vi "measurement_loop_template.vi"(8 "error in (no error)":errorcluster, 9 "Hardware.lvclass":refnum<class "Hardware.lvclass">, 10 "Notifiers":T2, 11 "Message Queues":T1) -> (0 "error out":errorcluster)   [LabVIEW 2017]
uses:
  Notifiers/Notifiers.ctl
  Message Queue/All Message Queues.ctl
  Message Queue/Message Cluster.ctl
  hardware/Hardware.lvclass
  measurement_state.ctl
  Message Queue/Enqueue Message (Single).vi
  <vilib>/Utility/error.llb/Error Cluster From Error Code.vi
  <vilib>/ErrorRing/Error Ring.xnode
  Message Queue/Message Queue.lvlib
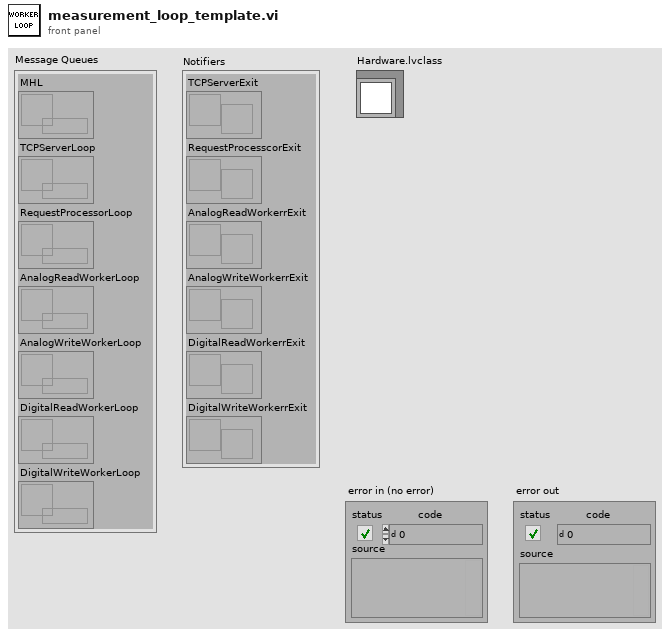
[diagram p1: front panel]
types:
  T1 = typedef "Message Queue.lvlib/All Message Queues.ctl" = cluster{"MHL":refnum<queue>, "TCPServerLoop":refnum<queue>, "RequestProcessorLoop":refnum<queue>, "AnalogReadWorkerLoop":refnum<queue>, "AnalogWriteWorkerLoop":refnum<queue>, "DigitalReadWorkerLoop":refnum<queue>, "DigitalWriteWorkerLoop":refnum<queue>}
  T2 = typedef "Notifiers.ctl" = cluster{"TCPServerExit":refnum<notifier>, "RequestProcesscorExit":refnum<notifier>, "AnalogReadWorkerrExit":refnum<notifier>, "AnalogWriteWorkerrExit":refnum<notifier>, "DigitalReadWorkerrExit":refnum<notifier>, "DigitalWriteWorkerrExit":refnum<notifier>}
  T3 = typedef "measurement_state.ctl" = enum16{"idle", "running"}
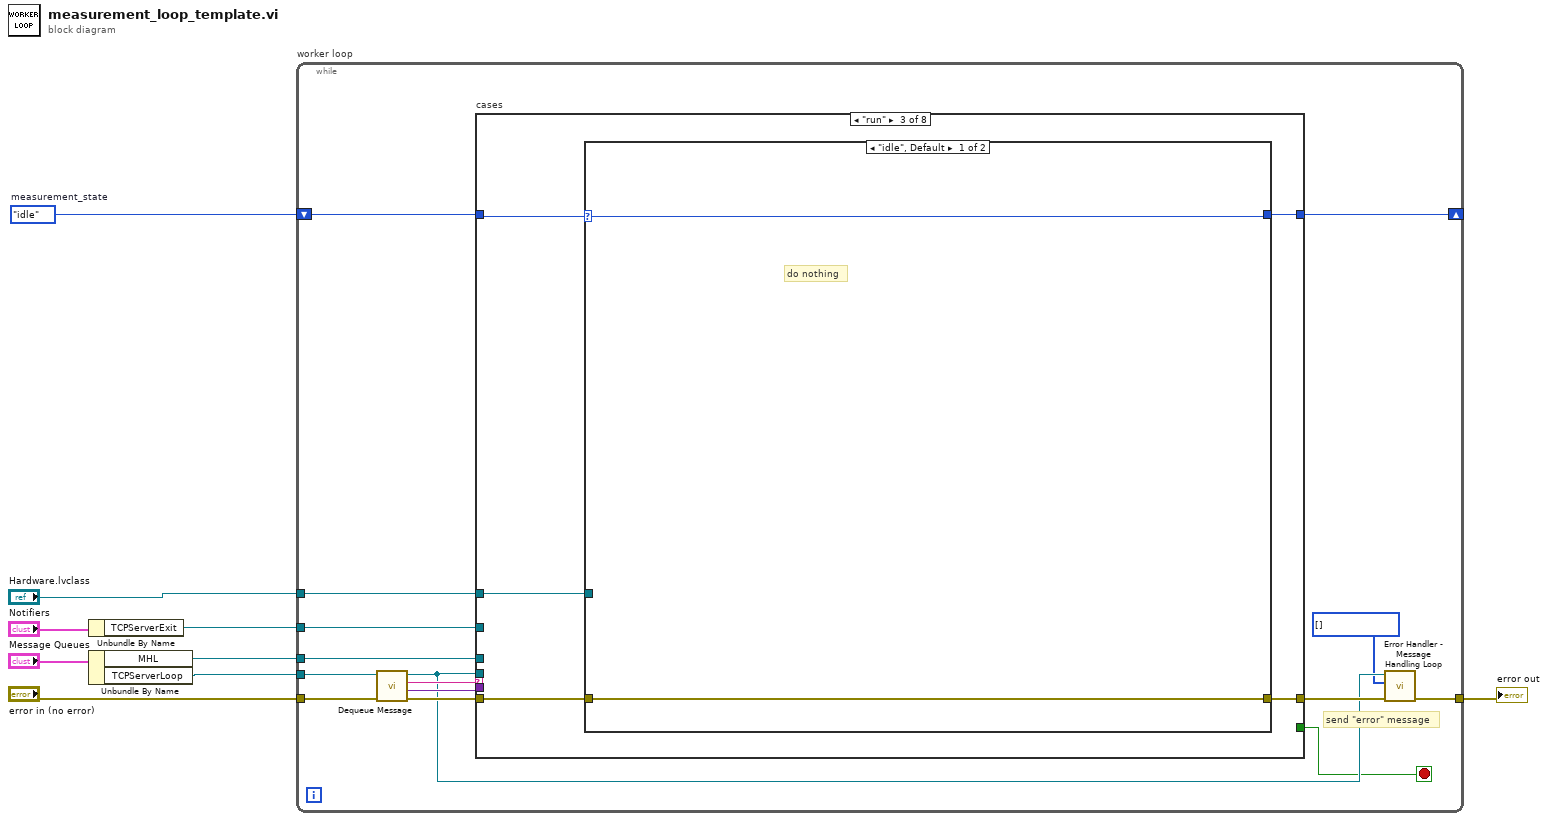
[diagram p0: block diagram]
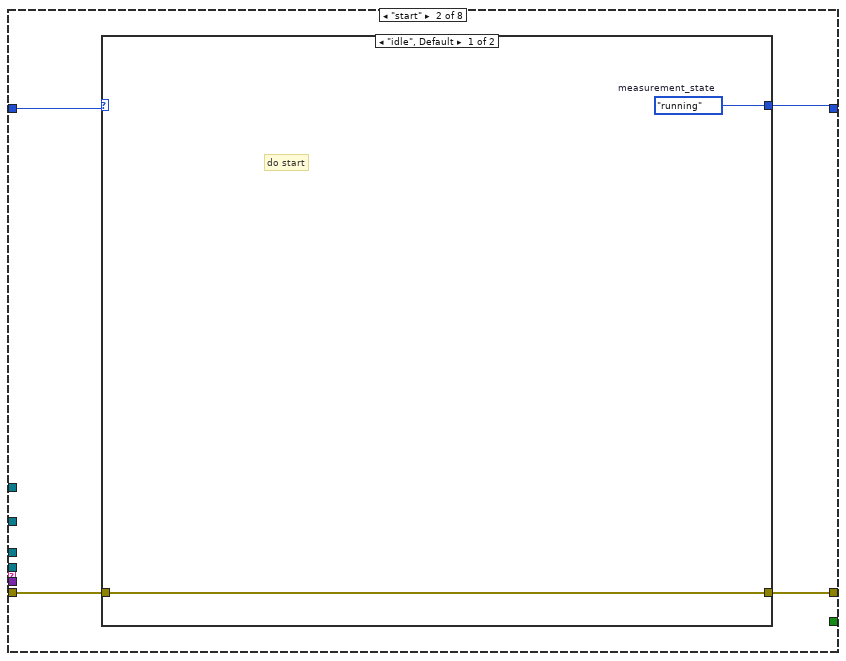
[diagram p3: hidden frame]
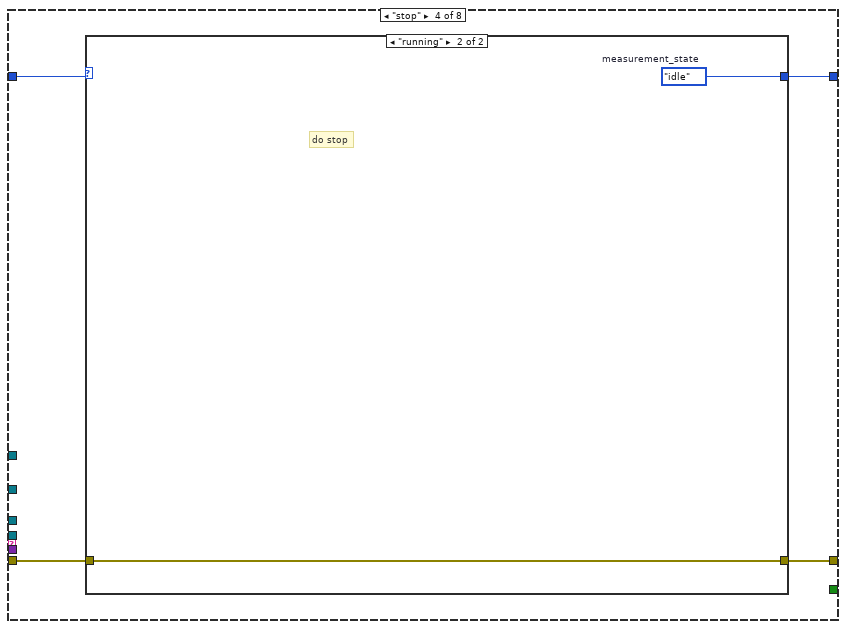
[diagram p6: hidden frame]
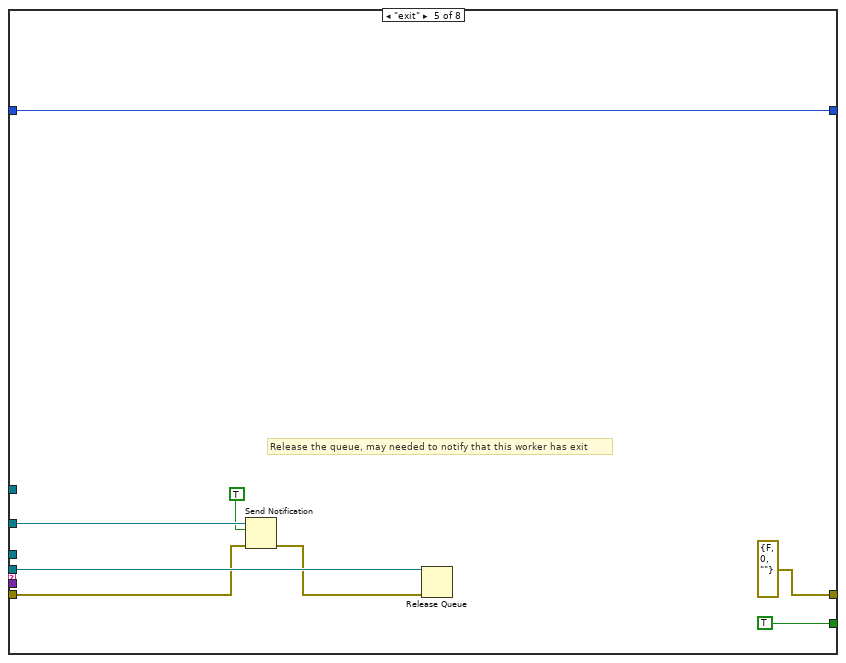
[diagram p8: hidden frame]
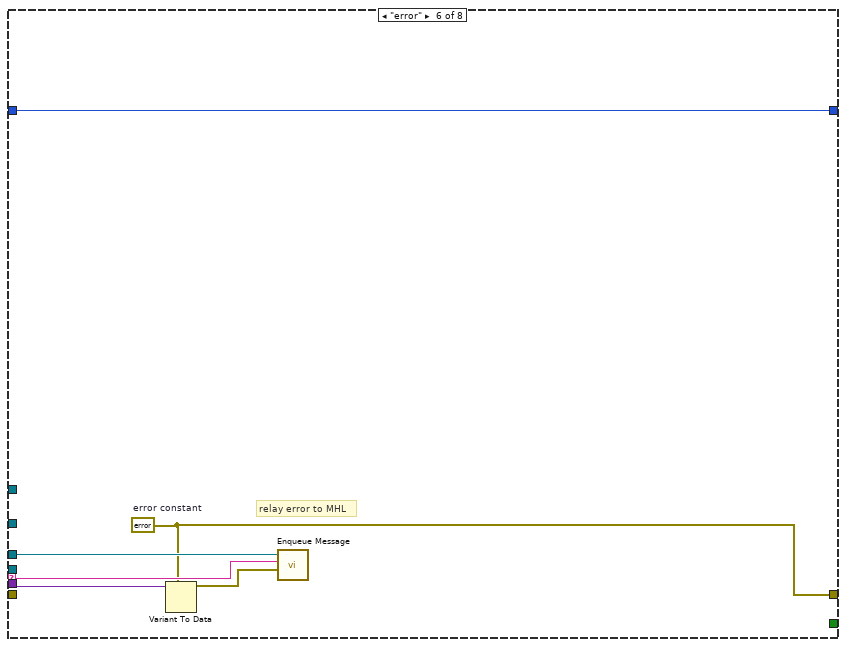
[diagram p9: hidden frame]
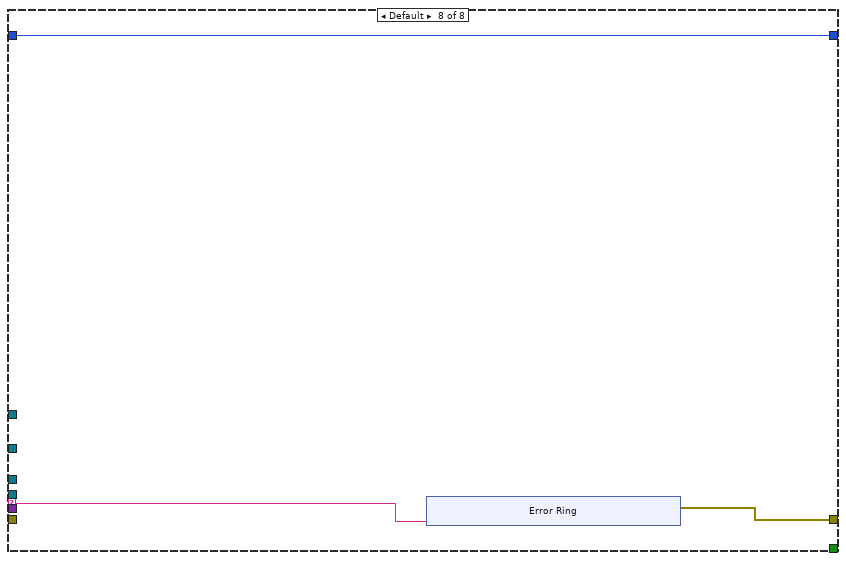
[diagram p11: hidden frame]
diagram:
  w1 = measurement_state."idle"  # measurement_state
  n1 = Unbundle By Name("Notifiers") -> ("TCPServerExit"=w3:refnum<notifier>)
  n2 = Unbundle By Name("Message Queues") -> ("MHL"=w5:refnum<queue>, "TCPServerLoop"=w6:refnum<queue>)
  n3 = while "worker loop" {
    tunnel: "error in (no error)" -> [w24]
    tunnel: [w19] -> w8
    tunnel: w6 -> [w15]
    tunnel: w5 -> [w14]
    tunnel: w3 -> [w13]
    tunnel: "Hardware.lvclass" -> [w12]
    shift-right: [w10] -> _
    shift-left: w1 -> [w11]
    stop <- w16 stop-if-true
    # "send \"error\" message"
    n4 = call "Dequeue Message.vi"("error in (no error)"=w24, "Message Queue"=w15) -> ("error out"=w23:errorcluster, "Message Data"=w21:variant, "Message"=w22:string, "dup Message Queue"=w18:refnum<queue>)  [unwired: 6 in]
    n5 = case "cases" shown="\"run\"" w22 {
      selector: w22 -> [_ _ _ _ _ w65 _ w70]
      tunnel: w23 -> [w26 w30 w36 w47 w55 _ w67 _]
      tunnel: [w26 w29 w35 w46 errorcluster {"status"=FALSE, "code"=0, "source"=""} ("error constant") w61 w67 w69] -> w20
      tunnel: w21 -> [_ _ _ _ _ w64 _ _]
      tunnel: w18 -> [_ _ _ _ w57 _ _ _]
      tunnel: [_ _ _ _ TRUE _ _ _] -> w16
      tunnel: w14 -> [_ _ _ _ _ w62 _ _]
      tunnel: w13 -> [_ _ _ _ w56 _ _ _]
      tunnel: w12 -> [_ _ w37 _ _ _ _ _]
      tunnel: w11 -> [w25 w28 w39 w45 w52 w60 w66 w68]
      tunnel: [w25 w27 w38 w44 w52 w60 w66 w68] -> w10
      frame "initiate" {
      }
      frame "start" {
        n6 = case shown="\"idle\", Default" w28 {
          selector: w28 -> [_ w33]
          tunnel: w30 -> [w31 w34]
          tunnel: [w31 w34] -> w29
          tunnel: [w32 w33] -> w27
          frame "idle", Default {
            w32 = measurement_state."running"  # measurement_state
            # "do start"
          }
          frame "running" {
            # "already running -> do nothing"
          }
        }
      }
      frame "run" {
        n7 = case shown="\"idle\", Default" w39 {
          selector: w39 -> [w41 w43]
          tunnel: [w41 w43] -> w38
          tunnel: w37 -> [_ _]
          tunnel: w36 -> [w40 w42]
          tunnel: [w40 w42] -> w35
          frame "idle", Default {
            # "do nothing"
          }
          frame "running" {
            # "do something since the the measurement is running"
          }
        }
      }
      frame "stop" {
        n8 = case shown="\"running\"" w45 {
          selector: w45 -> [w48 _]
          tunnel: w47 -> [w49 w51]
          tunnel: [w49 w51] -> w46
          tunnel: [w48 w50] -> w44
          frame "idle", Default {
            # "do nothing"
          }
          frame "running" {
            w50 = measurement_state."idle"  # measurement_state
            # "do stop"
          }
        }
      }
      frame "exit" {
        # "Release the queue, may needed to notify that this worker has exit"
        n9 = Send Notification(notification=TRUE, notifier=w56, error in (no error)=w55) -> (error out=w54:errorcluster)  [unwired: 1 out]
        n10 = Release Queue(queue=w57, error in (no error)=w54) -> ()  [unwired: 1 in, 3 out]
      }
      frame "error" {
        w61 = errorcluster {"status"=FALSE, "code"=0, "source"=""}  # error constant
        # "relay error to MHL"
        n11 = Variant To Data(type=w61, Variant=w64) -> (data=w63:errorcluster)  [unwired: 1 in, 1 out]
        n12 = call-poly "Enqueue Message.vi"("Message Data"=w63, "Message"=w65, "Message Queue"=w62) -> ()  [unwired: 7 in, 2 out]
      }
      frame "duplicate_me" {
      }
      frame Default {
        n13 = xnode "Error Ring"("parameter 0"=w70) -> ("error out"=w69:errorcluster)
      }
    }
    n14 = call "Error Handler - Message Handling Loop.vi"("error in (no error)"=w20, "Ignore Errors (Runtime)"=i32[] [], "Message Queue"=w18) -> ("dup error in"=w19:errorcluster)  [unwired: 7 in, 1 out]
  }
  "error out" <- w8
